vi "FTW-Menu-BuildLevel.vi"(0 "MenuRef":refnum<k9>, 5 "Menu Items":T1[](array[typedef]), 7 "Parent Tag (empty=root)":string, 11 "error in":errorcluster) -> (4 "MenuRef out":refnum<k9>, 15 "error out":errorcluster)   [LabVIEW 2014]
uses:
  FTW-Menu-Item.ctl
panel:
  # "Inputs"
  # "Outputs"
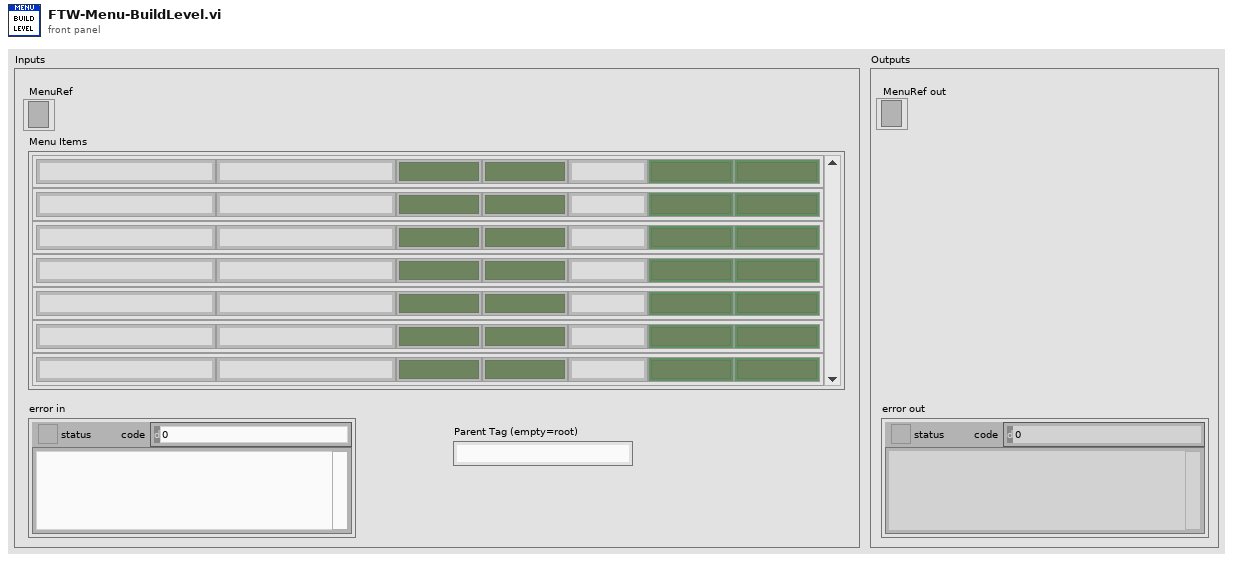
[diagram p1: front panel]
types:
  T1 = typedef "FTW-Menu-Item.ctl" = cluster{"Item Name":string, "Item Tag":string, "Checked":bool, "Enabled":bool, "Shortcut Key":string, "Shortcut+Ctrl":bool, "Shortcut+Shift":bool}
  T2 = cluster{"Shortcut+Shift":bool, "Shortcut+Ctrl":bool, "Shortcut Key":string}
  T3 = cluster{"Item Tag":string, cluster{"Shortcut+Shift":bool, "Shortcut+Ctrl":bool, "Shortcut Key":string}}
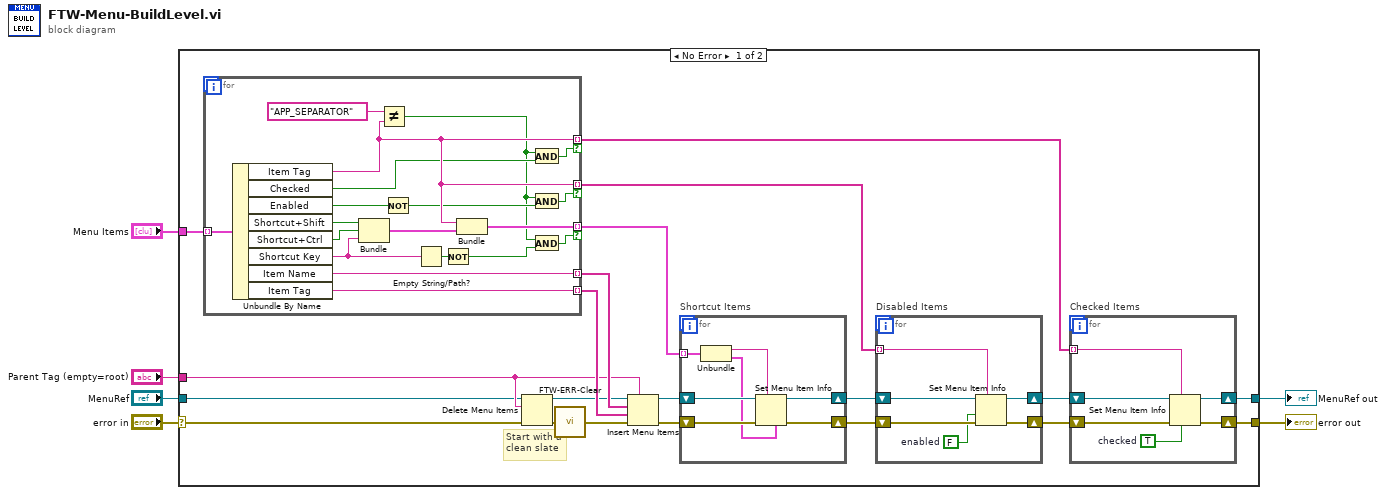
[diagram p0: block diagram]
diagram:
  n1 = case shown="No Error" "error in" {
    selector: "error in" -> [w9 w66]
    tunnel: "Menu Items" -> [w24 _]
    tunnel: "MenuRef" -> [w10 w65]
    tunnel: "Parent Tag (empty=root)" -> [w11 _]
    tunnel: [w13 w65] -> w3
    tunnel: [w12 w66] -> w2
    frame No Error {
      # "Start with a\nclean slate"
      n2 = for {
        tunnel: w24 -> [w64] mode=indexing
        tunnel: [w54] -> w14 mode=indexing if=w51
        tunnel: [w54] -> w17 mode=indexing if=w49
        tunnel: [w60] -> w23 mode=indexing
        tunnel: [w59] -> w22 mode=indexing
        tunnel: [w55] -> w21 mode=indexing if=w47
        n3 = Unbundle By Name(w64) -> ("Item Tag"=w54:string, "Checked"=w52:bool, "Enabled"=w61:bool, "Shortcut+Shift"=w63:bool, "Shortcut+Ctrl"=w62:bool, "Shortcut Key"=w58:string, "Item Name"=w60:string, "Item Tag"=w59:string)
        n4 = Bundle("Shortcut+Shift"=w63, "Shortcut+Ctrl"=w62, "Shortcut Key"=w58) -> (w56:T2)  [unwired: 1 in]
        n5 = Not Equal?(x="APP_SEPARATOR", y=w54) -> (x != y?=w48:bool)
        n6 = Not(x=w61) -> (.not. x?=w50:bool)
        n7 = Empty String/Path?(string/path=w58) -> (empty?=w57:bool)
        n8 = Not(x=w57) -> (.not. x?=w46:bool)
        n9 = Bundle("Item Tag"=w54, w56) -> (w55:T3)  [unwired: 1 in]
        n10 = And(x=w48, y=w52) -> (x .and. y?=w51:bool)
        n11 = And(x=w48, y=w50) -> (x .and. y?=w49:bool)
        n12 = And(x=w48, y=w46) -> (x .and. y?=w47:bool)
      }
      n13 = Delete Menu Items(6:w9, 8:w11, 9:w10) -> (0:w8:errorcluster, 3:w20:refnum<k9>)  [unwired: 1 in]
      n14 = call "FTW-ERR-Clear.vi"("error to snuff"=w8) -> ("no error"=w7:errorcluster)
      n15 = Insert Menu Items(5:w11, 6:w7, 7:w22, 8:w23, 9:w20) -> (0:w25:errorcluster, 3:w26:refnum<k9>)  [unwired: 1 in, 1 out]
      n16 = for "Shortcut Items" {
        shift-right: [w43] -> w19
        shift-left: w26 -> [w45]
        shift-right: [w42] -> w18
        shift-left: w25 -> [w44]
        tunnel: w21 -> [w41] mode=indexing
        n17 = Unbundle(w41) -> ("Item Tag"=w40:string, w39:T2)
        n18 = Set Menu Item Info(4:w39, 7:w40, 8:w44, 11:w45) -> (0:w42:errorcluster, 3:w43:refnum<k9>)  [unwired: 3 in]
      }
      n19 = for "Disabled Items" {
        shift-right: [w36] -> w16
        shift-left: w19 -> [w38]
        shift-right: [w35] -> w15
        shift-left: w18 -> [w37]
        tunnel: w17 -> [w34] mode=indexing
        w33 = FALSE  # enabled
        n20 = Set Menu Item Info(7:w34, 8:w37, 9:w33, 11:w38) -> (0:w35:errorcluster, 3:w36:refnum<k9>)  [unwired: 3 in]
      }
      n21 = for "Checked Items" {
        shift-right: [w30] -> w13
        shift-left: w16 -> [w32]
        shift-right: [w29] -> w12
        shift-left: w15 -> [w31]
        tunnel: w14 -> [w28] mode=indexing
        w27 = TRUE  # checked
        n22 = Set Menu Item Info(6:w27, 7:w28, 8:w31, 11:w32) -> (0:w29:errorcluster, 3:w30:refnum<k9>)  [unwired: 3 in]
      }
    }
    frame Error {
    }
  }
  "error out" <- w2
  "MenuRef out" <- w3
